vi "Write Display Name.vi"(8 "error in (no error)":errorcluster, 10 "Display Name":string, 11 "Task in":refnum<class "Task.lvclass">) -> (0 "error out":errorcluster, 3 "Task out":refnum<class "Task.lvclass">)   [LabVIEW 2017, in "Task Interface.lvlib" / "Task.lvclass"]
uses:
  Task.lvclass
  Task.lvclass/Task.ctl
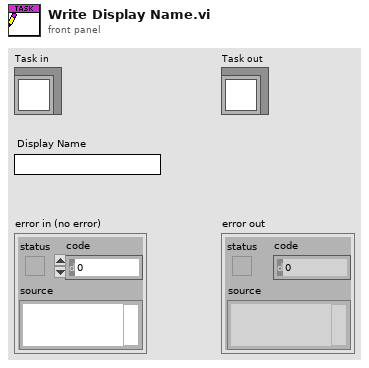
[diagram p1: front panel]
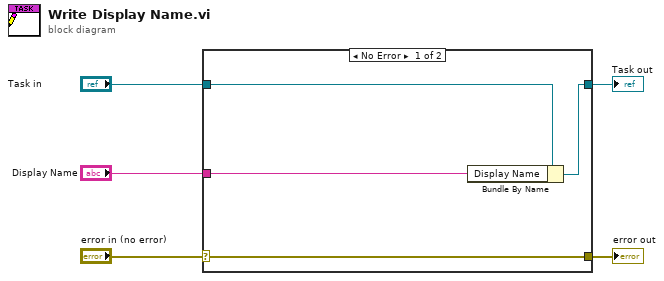
[diagram p0: block diagram]
diagram:
  n1 = case shown="No Error" "error in (no error)" {
    selector: "error in (no error)" -> [w9 w10]
    tunnel: [w9 w10] -> w4
    tunnel: [w7 w11] -> w2
    tunnel: "Task in" -> [w8 w11]
    tunnel: "Display Name" -> [w6 _]
    frame No Error {
      n2 = Bundle By Name(cluster=w8, "Display Name"=w6) -> (w7:refnum<class "Task.lvclass">)
    }
    frame Error {
    }
  }
  "error out" <- w4
  "Task out" <- w2
